vi "NormalizeAngle.vi"(1 "Angle (rad)":dbl) -> (0 "angle (between pi and -pi)":dbl(knob) scale=0.0..10.0)   [LabVIEW 2015]
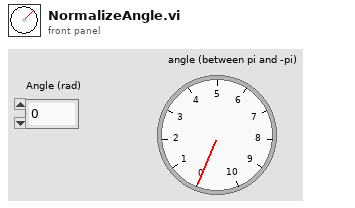
[diagram p1: front panel]
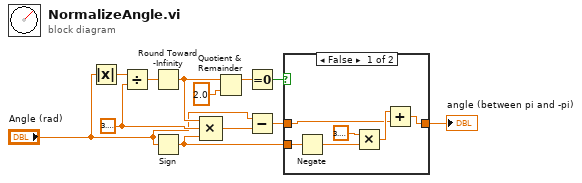
[diagram p0: block diagram]
diagram:
  w9 = 3.141592653589793
  n1 = Absolute Value(x="Angle (rad)") -> (abs(x)=w12:dbl)
  n2 = Divide(x=w12, y=w9) -> (x/y=w11:dbl)
  n3 = Round Toward -Infinity(1:w11) -> (0:w8:dbl)
  n4 = Sign(1:"Angle (rad)") -> (0:w2:dbl)
  n5 = Compound Arithmetic op=MULTIPLY(w8, w9, w2) -> (w10:dbl)
  n6 = Quotient & Remainder(x=w8, y=2.0) -> (x-y*floor(x/y)=w6:dbl)  [unwired: 1 out]
  n7 = Equal To 0?(x=w6) -> (x = 0?=w4:bool)
  n8 = Subtract(x="Angle (rad)", y=w10) -> (x-y=w3:dbl)
  n9 = case shown="False" w4 {
    tunnel: [w13 w19] -> w1
    tunnel: w3 -> [w14 w19]
    tunnel: w2 -> [w15 _]
    frame False {
      n10 = Negate(x=w15) -> (-x=w17:dbl)
      n11 = Multiply(x=3.141592653589793, y=w17) -> (x*y=w16:dbl)
      n12 = Add(x=w16, y=w14) -> (x+y=w13:dbl)
    }
    frame True {
    }
  }
  "angle (between pi and -pi)" <- w1
